vi "MPExxx_set_arm.vi"(2 "error in (no error)":errorcluster, 3 "ARM":bool, 4 "VISA session":refnum<visa-resource-name>) -> (0 "error out":errorcluster, 1 "dup VISA session":refnum<visa-resource-name>)   [LabVIEW 2012]
doc: "This VI form selects between the modes of operation. There are two modes of operation for the power supply: normal mode and auto sequence mode. Normal mode energizes the current parameters of the supply until stopped. Auto sequence mode sequentially steps through the memory updating the supply's parameters as it increments. Each memory location contains the voltage set point, current set point, over voltage trip, over current trip, and period. The period parameter specifies the time period for operating at the memory location when auto sequence operation is deployed. When enabled, the ARM light lights on the on the front panel."
uses:
  MPExxx Globals.gbl
panel:
  # "MAGNA-POWER"
  # "Electronics"
  # "ON"
  # "OFF"
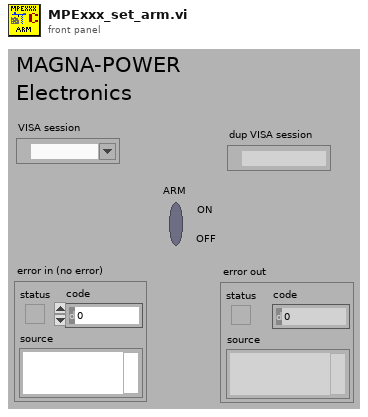
[diagram p1: front panel]
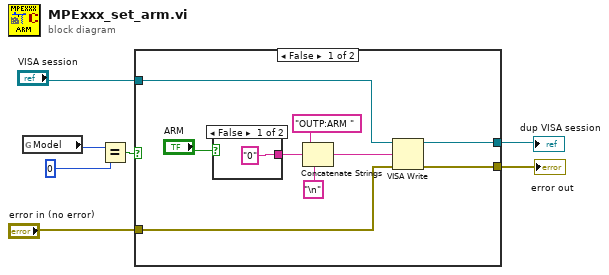
[diagram p0: block diagram]
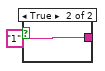
[diagram p2: hidden frame]
diagram:
  n1 = global read "MPExxx Globals.gbl" "Model"() -> (w5:u8)
  n2 = Equal?(x=w5, y=0) -> (x = y?=w7:bool)
  n3 = case shown="False" w7 {
    tunnel: "VISA session" -> [w12 w20]
    tunnel: "error in (no error)" -> [w11 w19]
    tunnel: [w9 w20] -> w2
    tunnel: [w8 w19] -> w1
    frame False {
      n4 = case shown="False" "ARM" {
        tunnel: ["0" "1"] -> w15
        frame False {
        }
        frame True {
        }
      }
      n5 = Concatenate Strings("OUTP:ARM ", w15, "\n") -> (w10:string)
      n6 = VISA Write(VISA resource name=w12, write buffer=w10, error in (no error)=w11) -> (VISA resource name out=w9:refnum<visa-resource-name>, error out=w8:errorcluster)  [unwired: 1 out]
    }
    frame True {
    }
  }
  "error out" <- w1
  "dup VISA session" <- w2
